vi "Start FPGA.vi"(8 "error in (no error)":errorcluster, 10 "Master Configuration":T2={"Epics Configuration"={"DIN1 Mask Out1"=[], "# Samples Post Trig"=5, "Armed"=FALSE, "ADC Mask"=[], "ADC Max Threshold"=[], "ADC Min Threshold"=[], "DIN Mask 2"=[], "DIN1 Mask Out2"=[], "DIN1 Mask Out3"=[], "DIN1 Mask Out4"=[], "Out3 Armed"=FALSE, "Out1 Armed"=FALSE, "Out4 Armed"=FALSE, "Out2 Armed"=FALSE}, "Epics Configuration File"="/EpicsConfig.cfg", "Number of Channels"=0, "Data rate"=0, "PM Buffer Size"=0}, 11 "FPGA VI Reference":T1) -> (0 "error out":errorcluster, 3 "FPGA VI Reference":T1)   [LabVIEW 2014]
uses:
  controls/Master Configuration.ctl
  controls/EPICS Configuration.ctl
  controls/FPGA VI Reference.ctl
  <vilib>/FPGAPlugInAG/Dynamic/niLvFpga_Reset_Dynamic.vi
  <vilib>/FPGAPlugInAG/Dynamic/niLvFpga_Run_Dynamic.vi
  <vilib>/Utility/error.llb/Error Cluster From Error Code.vi
  <vilib>/RVI Host/nirviSupport.llb/nirviErrorClusterFromErrorCode.vi
  <vilib>/rvi/errors/niLvFpgaAdjustHostInterfaceError.vi
  <vilib>/rvi/interface/common/niFpgaWaitOnOcc.vi
  <vilib>/rvi/interface/nirviMethod/nirviMethod.xnode
  <vilib>/rvi/interface/nirviReadWriteControl/nirviReadWriteControl.xnode
  <vilib>/rvi/interface/nirviMethod/StockFPGA_InlinedMethodWaitForSingleIRQ.vi
  <vilib>/FPGAPlugInAG/Dynamic/niLvFpga_WaitOnIrq_Dynamic.vi
  <vilib>/FPGAPlugInAG/Dynamic/niLvFpga_AcknowledgeIrq_Dynamic.vi
  <vilib>/FPGAPlugInAG/Dynamic/niLvFpga_ConfigureFifo_Dynamic.vi
  <vilib>/rvi/errors/niLvFpgaMergeErrorWithErrorCode.vi
  NiFpgaLv.dll
  <vilib>/rvi/interface/Simulation/niFpgaSimulationCallBeginRW.vi
panel:
  out "Actual Depth":u32
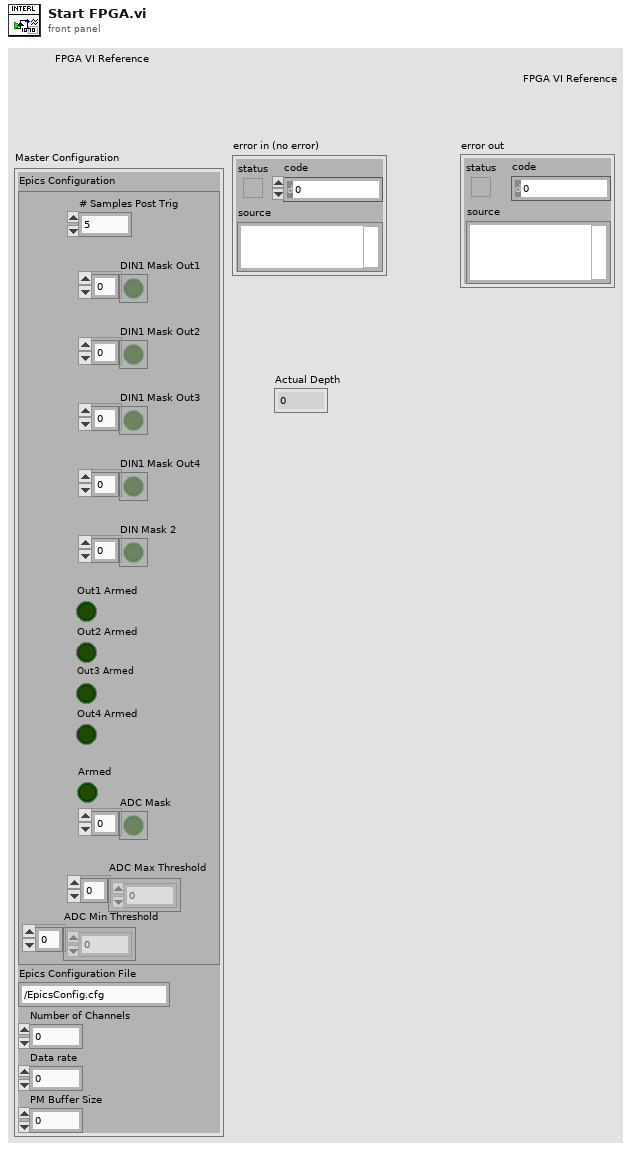
[diagram p1: front panel]
types:
  T1 = typedef "FPGA VI Reference.ctl" = refnum<k20>
  T2 = typedef "Master Configuration.ctl" = cluster{"Epics Configuration":T3, "Epics Configuration File":string, "Number of Channels":u8, "Data rate":u32, "PM Buffer Size":u32}
  T3 = typedef "EPICS Configuration.ctl" = cluster{"DIN1 Mask Out1":bool[], "# Samples Post Trig":u32, "Armed":bool, "ADC Mask":bool[], "ADC Max Threshold":dbl[], "ADC Min Threshold":dbl[], "DIN Mask 2":bool[], "DIN1 Mask Out2":bool[], "DIN1 Mask Out3":bool[], "DIN1 Mask Out4":bool[], "Out3 Armed":bool, "Out1 Armed":bool, "Out4 Armed":bool, "Out2 Armed":bool}
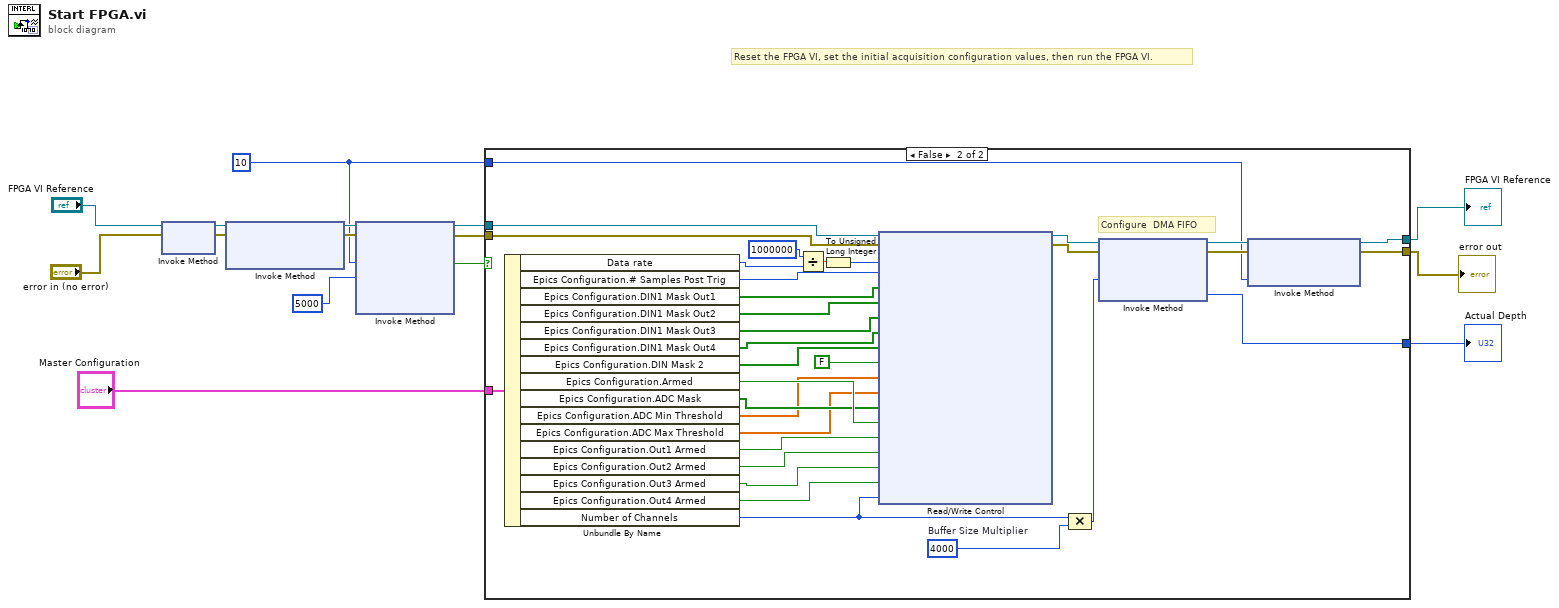
[diagram p0: block diagram]
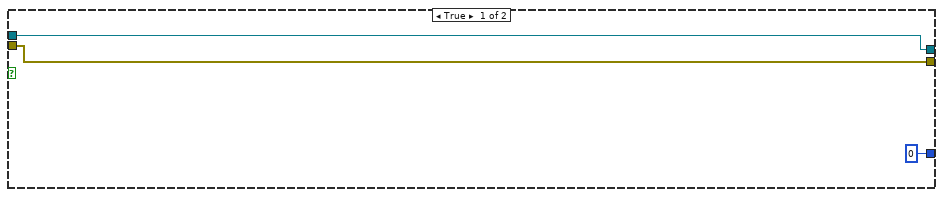
[diagram p2: hidden frame]
diagram:
  w2 = 10
  # "Reset the FPGA VI, set the initial acquisition configuration values, then run the FPGA VI."
  n1 = xnode "Invoke Method"("FPGA VI Reference In"="FPGA VI Reference", "error in"="error in (no error)") -> ("FPGA VI Reference Out"=w6:T1, "error out"=w5:errorcluster)
  n2 = xnode "Invoke Method"("FPGA VI Reference In"=w6, "error in"=w5) -> ("FPGA VI Reference Out"=w4:T1, "error out"=w3:errorcluster)  [unwired: 1 in]
  n3 = xnode "Invoke Method"("FPGA VI Reference In"=w4, "error in"=w3, "IRQ Number(s)"=w2, "Timeout (ms)"=5000) -> ("FPGA VI Reference Out"=w9:T1, "error out"=w8:errorcluster, "Timed Out"=w7:bool)  [unwired: 1 out]
  n4 = case shown="False" w7 {
    tunnel: [w17 w37] -> w15
    tunnel: [w18 w36] -> w14
    tunnel: "Master Configuration" -> [_ w51]
    tunnel: w9 -> [w18 w41]
    tunnel: w8 -> [w17 w40]
    tunnel: w2 -> [_ w35]
    tunnel: [u32 0 ("Actual Depth") w34] -> w1
    frame True {
    }
    frame False {
      w48 = 4000  # Buffer Size Multiplier
      # "Configure  DMA FIFO"
      n5 = Unbundle By Name(w51) -> ("Data rate"=w46:u32, "Epics Configuration.# Samples Post Trig"=w43:u32, "Epics Configuration.DIN1 Mask Out1"=w27:bool[], "Epics Configuration.DIN1 Mask Out2"=w26:bool[], "Epics Configuration.DIN1 Mask Out3"=w24:bool[], "Epics Configuration.DIN1 Mask Out4"=w25:bool[], "Epics Configuration.DIN Mask 2"=w28:bool[], "Epics Configuration.Armed"=w33:bool, "Epics Configuration.ADC Mask"=w31:bool[], "Epics Configuration.ADC Min Threshold"=w30:dbl[], "Epics Configuration.ADC Max Threshold"=w29:dbl[], "Epics Configuration.Out1 Armed"=w19:bool, "Epics Configuration.Out2 Armed"=w20:bool, "Epics Configuration.Out3 Armed"=w21:bool, "Epics Configuration.Out4 Armed"=w22:bool, "Number of Channels"=w23:u8)
      n6 = Divide(x=1000000 ("y"), y=w46) -> (x/y=w44:dbl)
      n7 = To Unsigned Long Integer(number=w44) -> (unsigned 32bit integer=w32:u32)
      n8 = xnode "Read/Write Control"("FPGA VI Reference In"=w41, "error in"=w40, "Sample Period (uSec)"=w32, "Number samples after trigger"=w43, "DIN1 Mask Out1"=w27, "DIN1 Mask Out2"=w26, "DIN1 Mask Out3"=w24, "DIN1 Mask Out4"=w25, "DIN Mask Mod4"=w28, "Data Acq Stop"=FALSE, "ADC Threshold min value"=w30, "ADC Threshold max value"=w29, "ADC Mask"=w31, "Interlock on"=w33, "Out1 Armed"=w19, "Out2 Armed"=w20, "Out3 Armed"=w21, "Out4 Armed"=w22, "Number of Channels"=w23) -> ("FPGA VI Reference Out"=w50:T1, "error out"=w49:errorcluster)
      n9 = Compound Arithmetic op=MULTIPLY(w23, w48) -> (w47:i32)
      n10 = xnode "Invoke Method"("FPGA VI Reference In"=w50, "error in"=w49, "Requested Depth"=w47) -> ("FPGA VI Reference Out"=w39:T1, "error out"=w38:errorcluster, "Actual Depth"=w34:u32)
      n11 = xnode "Invoke Method"("FPGA VI Reference In"=w39, "error in"=w38, "IRQ Number(s)"=w35) -> ("FPGA VI Reference Out"=w36:T1, "error out"=w37:errorcluster)
    }
  }
  "error out" <- w15
  "FPGA VI Reference" <- w14
  "Actual Depth" <- w1
